vi "full teleop + start button.vi"() -> ()   [LabVIEW 2010, in "Tank Robot.lvrbt"]
uses:
  Tank Robot.lvrbt
  <vilib>/NXT/Subs/LVHSConnector.ctl
  <vilib>/NXT/NXTIO Xnodes/AddressXNode/NXTIOAddress.xnode
  <vilib>/NXT/Subs/MotorXNode.Servo Type.ctl
  <vilib>/NXT/Subs/MotorXNode.1Servo.ctl
  <vilib>/NXT/NXTIO Xnodes/NXTIOXNode/NXTIO.xnode
  <vilib>/NXT/Subs/MotorXNode.DC Motor Type.ctl
  <vilib>/NXT/Subs/MotorXNode.2DCMotor.ctl
  <vilib>/NXT/NXTIO Xnodes/NXTIONodeSubVIs/TETRIX IO Move Servos.vi
  <vilib>/FTC/FTC Calculate Drive Power - Tank.vi
  <vilib>/NXT/NXTIO Xnodes/NXTIONodeSubVIs/TETRIX IO Move DC Motors.vi
  <vilib>/NXT/Dual Mode Library/Display/drawNumber_float.vi
panel:
  out "Default":bool
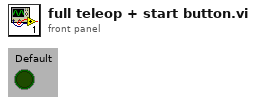
[diagram p1: front panel]
types:
  T1 = typedef "LVHSConnector.ctl" = cluster{"Hardware":string, "Flattened String":string}
  T2 = typedef "FTC ControllerState.ctl" = cluster{"Left X":i8, "Left Y":i8, "Right X":i8, "Right Y":i8, "Button Encoding 9-12":u8, "Button Encoding 1-8":u8, "POV":T3}
  T3 = typedef "FTC POVState.ctl" = i8
  T4 = typedef "FTC ButtonState.ctl" = cluster{"Button 1":bool, "Button 2":bool, "Button 3":bool, "Button 4":bool, "Button 5":bool, "Button 6":bool, "Button 7":bool, "Button 8":bool, "Button 9":bool, "Button 10":bool, "Button 11":bool, "Button 12":bool, "POV":T3}
  T5 = typedef "MotorXNode.Servo Type.ctl" = enum16{"Servo"}
  T6 = typedef "MotorXNode.DC Motor Type.ctl" = enum16{"DC Motor"}
  T7 = cluster{"DC Motor":T6, "Address":i16, "Address":i16}
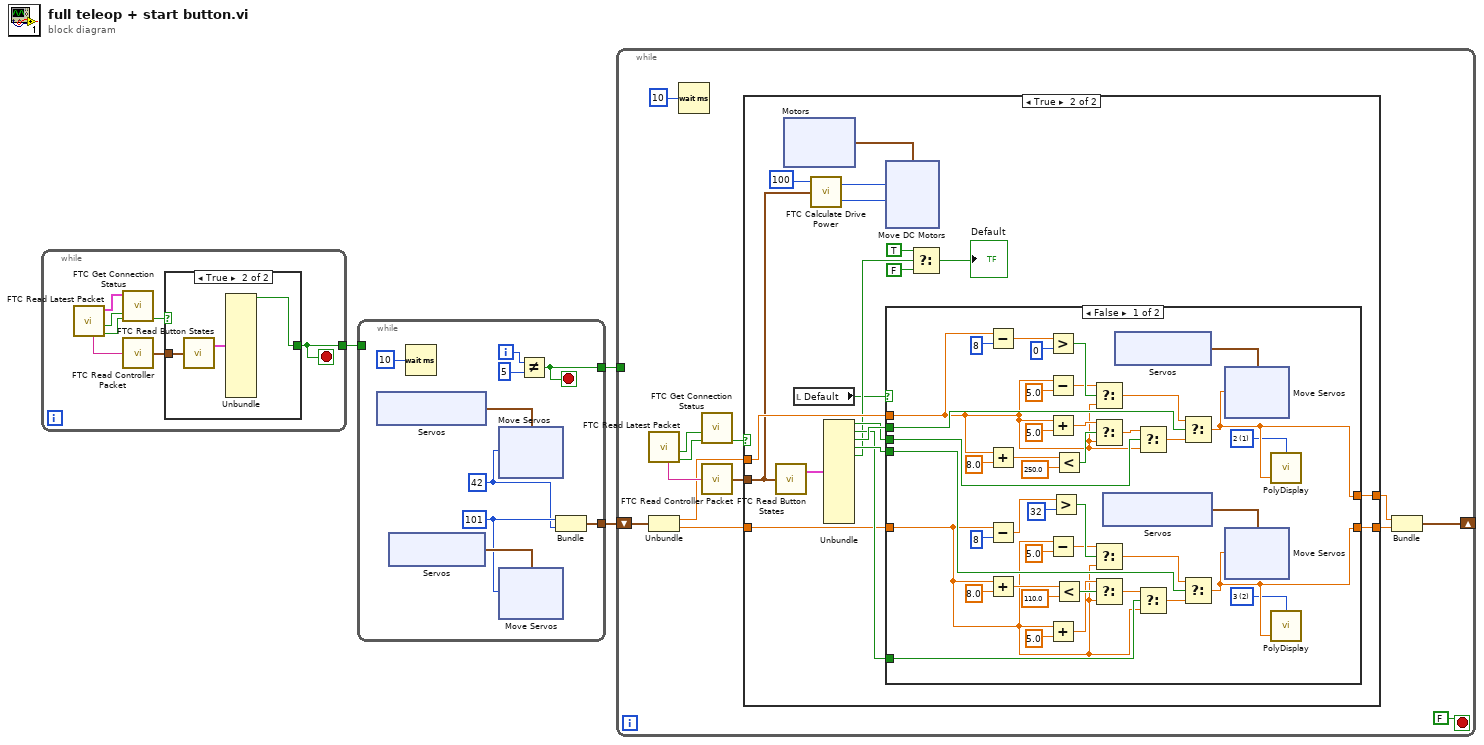
[diagram p0: block diagram]
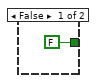
[diagram p2: hidden frame]
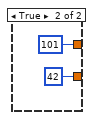
[diagram p4: hidden frame]
diagram:
  n1 = while {
    tunnel: [w4] -> w1
    stop <- w4 stop-if-true
    n2 = call <vilib>:"FTC Read Latest Packet.vi"() -> ("Packet Received?"=w10:bool, "Stopped?"=w9:bool, "NXT"=w8:T1, "Controller 1"=w6:string)  [unwired: 6 in, 2 out]
    n3 = call <vilib>:"FTC Get Connection Status.vi"("Packet Received?"=w10, "Stopped?"=w9, "NXT"=w8) -> ("Online?"=w7:bool)  [unwired: 5 in, 2 out]
    n4 = call <vilib>:"FTC Read Controller Packet.vi"("Packet"=w6) -> ("Controller State"=w5:T2)  [unwired: 4 in]
    n5 = case shown="True" w7 {
      tunnel: w5 -> [_ w14]
      tunnel: [FALSE w12] -> w4
      frame False {
      }
      frame True {
        n6 = call <vilib>:"FTC Read Button States.vi"("Controller State"=w14) -> ("Button States"=w13:T4)  [unwired: 2 in, 1 out]
        n7 = Unbundle(w13) -> ("Button 1"=w12:bool)  [unwired: 12 out]
      }
    }
  }
  n8 = while {
    tunnel: [w20] -> w3
    tunnel: [w15] -> w2
    tunnel: w1 -> [_]
    i -> [w23]
    stop <- w20 stop-if-true
    w16 = u8 42 ("Position 1")
    w17 = u8 101 ("Position 1")
    n9 = xnode "Servos"() -> ("Servo"=w18:cluster{"Servo":T5, "Address":i16})
    n10 = xnode "Servos"() -> ("Servo"=w19:cluster{"Servo":T5, "Address":i16})
    n11 = Wait (ms)(milliseconds to wait=u32 10) -> ()  [unwired: 1 out]
    n12 = xnode "Move Servos"("Position 1"=w16, "Servos"=w18) -> ()  [unwired: 1 in, 1 out]
    n13 = xnode "Move Servos"("Position 1"=w17, "Servos"=w19) -> ()  [unwired: 1 in, 1 out]
    n14 = Not Equal?(x=w23, y=5) -> (x != y?=w20:bool)
    n15 = Bundle("Position 1"=w17, "Position 1"=w16) -> (w15:cluster{"Position 1":u8, "Position 1":u8})  [unwired: 1 in]
  }
  n16 = while {
    tunnel: w3 -> [_]
    shift-right: [w42] -> _
    shift-left: w2 -> [w47]
    stop <- FALSE stop-if-true
    n17 = call <vilib>:"FTC Read Latest Packet.vi"() -> ("Packet Received?"=w51:bool, "Stopped?"=w52:bool, "Controller 1"=w49:string)  [unwired: 6 in, 3 out]
    n18 = Unbundle(w47) -> ("Position 1"=w46:dbl, "Position 1"=w45:dbl)
    n19 = Wait (ms)(milliseconds to wait=u32 10) -> ()  [unwired: 1 out]
    n20 = call <vilib>:"FTC Get Connection Status.vi"("Packet Received?"=w51, "Stopped?"=w52) -> ("Online?"=w50:bool)  [unwired: 6 in, 2 out]
    n21 = call <vilib>:"FTC Read Controller Packet.vi"("Packet"=w49) -> ("Controller State"=w48:T2)  [unwired: 4 in]
    n22 = case shown="True" w50 {
      tunnel: w48 -> [_ w67]
      tunnel: w46 -> [w56 w73]
      tunnel: w45 -> [w55 w69]
      tunnel: [w56 w72] -> w44
      tunnel: [w55 w68] -> w43
      frame False {
      }
      frame True {
        n23 = call <vilib>:"FTC Read Button States.vi"("Controller State"=w67) -> ("Button States"=w62:T4)  [unwired: 2 in, 1 out]
        n24 = xnode "Motors"() -> ("DC Motor"=w65:T7)
        n25 = local read "Default"() -> (w57:bool)
        n26 = call-poly <vilib>:"FTC Calculate Drive Power.vi"("Controller State"=w67, "Power Level (50)"=i8 100) -> ("Right Motor Power"=w63:i8, "Left Motor Power"=w64:i8)  [unwired: 2 in]
        n27 = Unbundle(w62) -> ("Button 1"=w74:bool, "Button 2"=w70:bool, "Button 3"=w75:bool, "Button 4"=w71:bool, "Button 5"=w61:bool)  [unwired: 8 out]
        n28 = xnode "Move DC Motors"("Power/Speed 2"=w63, "Power/Speed 1"=w64, "Motors"=w65) -> ()  [unwired: 1 in, 1 out]
        n29 = case shown="False" w57 {
          tunnel: w75 -> [w109 _]
          tunnel: w74 -> [w108 _]
          tunnel: w73 -> [w100 _]
          tunnel: [w79 101] -> w72
          tunnel: w71 -> [w82 _]
          tunnel: w70 -> [w81 _]
          tunnel: w69 -> [w80 _]
          tunnel: [w77 42] -> w68
          frame False {
            w76 = i16 2 items=["1", "2", "3", "4", "5", "6", "7", "8"] ("Line")
            w78 = i16 1 items=["1", "2", "3", "4", "5", "6", "7", "8"] ("Line")
            n30 = Subtract(x=w100, y=u8 8) -> (x-y=w115:dbl)
            n31 = Add(x=w100, y=8.0) -> (x+y=w106:dbl)
            n32 = Subtract(x=w80, y=u8 8) -> (x-y=w96:dbl)
            n33 = Add(x=w80, y=8.0) -> (x+y=w89:dbl)
            n34 = Greater?(x=w115, y=u8 0) -> (0:w113:bool)
            n35 = Subtract(x=w100, y=5.0) -> (x-y=w112:dbl)
            n36 = Add(x=w100, y=5.0) -> (x+y=w103:dbl)
            n37 = Subtract(x=w80, y=5.0) -> (x-y=w93:dbl)
            n38 = Add(x=w80, y=5.0) -> (x+y=w86:dbl)
            n39 = Greater?(x=w96, y=u8 32) -> (0:w94:bool)
            n40 = Less?(x=w106, y=250.0) -> (x < y?=w104:bool)
            n41 = Less?(x=w89, y=110.0) -> (x < y?=w87:bool)
            n42 = Select(t=w112, s=w113, f=w100) -> (s? t:f=w110:dbl)
            n43 = Select(t=w103, s=w104, f=w100) -> (s? t:f=w101:dbl)
            n44 = Select(t=w93, s=w94, f=w80) -> (s? t:f=w91:dbl)
            n45 = Select(t=w86, s=w87, f=w80) -> (s? t:f=w84:dbl)
            n46 = xnode "Servos"() -> ("Servo"=w98:cluster{"Servo":T5, "Address":i16})
            n47 = xnode "Servos"() -> ("Servo"=w117:cluster{"Servo":T5, "Address":i16})
            n48 = Select(t=w101, s=w108, f=w100) -> (s? t:f=w99:dbl)
            n49 = Select(t=w84, s=w81, f=w80) -> (s? t:f=w83:dbl)
            n50 = Select(t=w110, s=w109, f=w99) -> (s? t:f=w79:dbl)
            n51 = Select(t=w91, s=w82, f=w83) -> (s? t:f=w77:dbl)
            n52 = xnode "Move Servos"("Position 1"=w79, "Servos"=w117) -> ()  [unwired: 1 in, 1 out]
            n53 = xnode "Move Servos"("Position 1"=w77, "Servos"=w98) -> ()  [unwired: 1 in, 1 out]
            n54 = call-poly <vilib>:"PolyDisplay.vi"("number"=w79, "Line"=w78) -> ()  [unwired: 2 in, 1 out]
            n55 = call-poly <vilib>:"PolyDisplay.vi"("number"=w77, "Line"=w76) -> ()  [unwired: 2 in, 1 out]
          }
          frame True {
          }
        }
        n56 = Select(t=TRUE, s=w61, f=FALSE) -> (s? t:f=→"Default":bool)
      }
    }
    n57 = Bundle("Position 1"=w44, "Position 1"=w43) -> (w42:cluster{"Position 1":dbl, "Position 1":dbl})  [unwired: 1 in]
  }
